vi "DependencyChecker.vi"() -> ()   [LabVIEW 2020]
uses:
  <vilib>/Utility/lvfile.llb/LVFileType.ctl
  FileDependencyType.ctl
  <vilib>/Utility/lvfile.llb/FT_FileTypes.ctl
  <vilib>/Utility/lvfile.llb/NI_FileType.lvlib
panel:
  out "size(s)":i32
  out "Files":map{path, T1}(c390)
  out "File Path 2":path
  out "Linker:Read Info From File":T4(array[cluster])
  in  "File Path":path=path "C:/Projects/DesignPatterns/Decorator1"
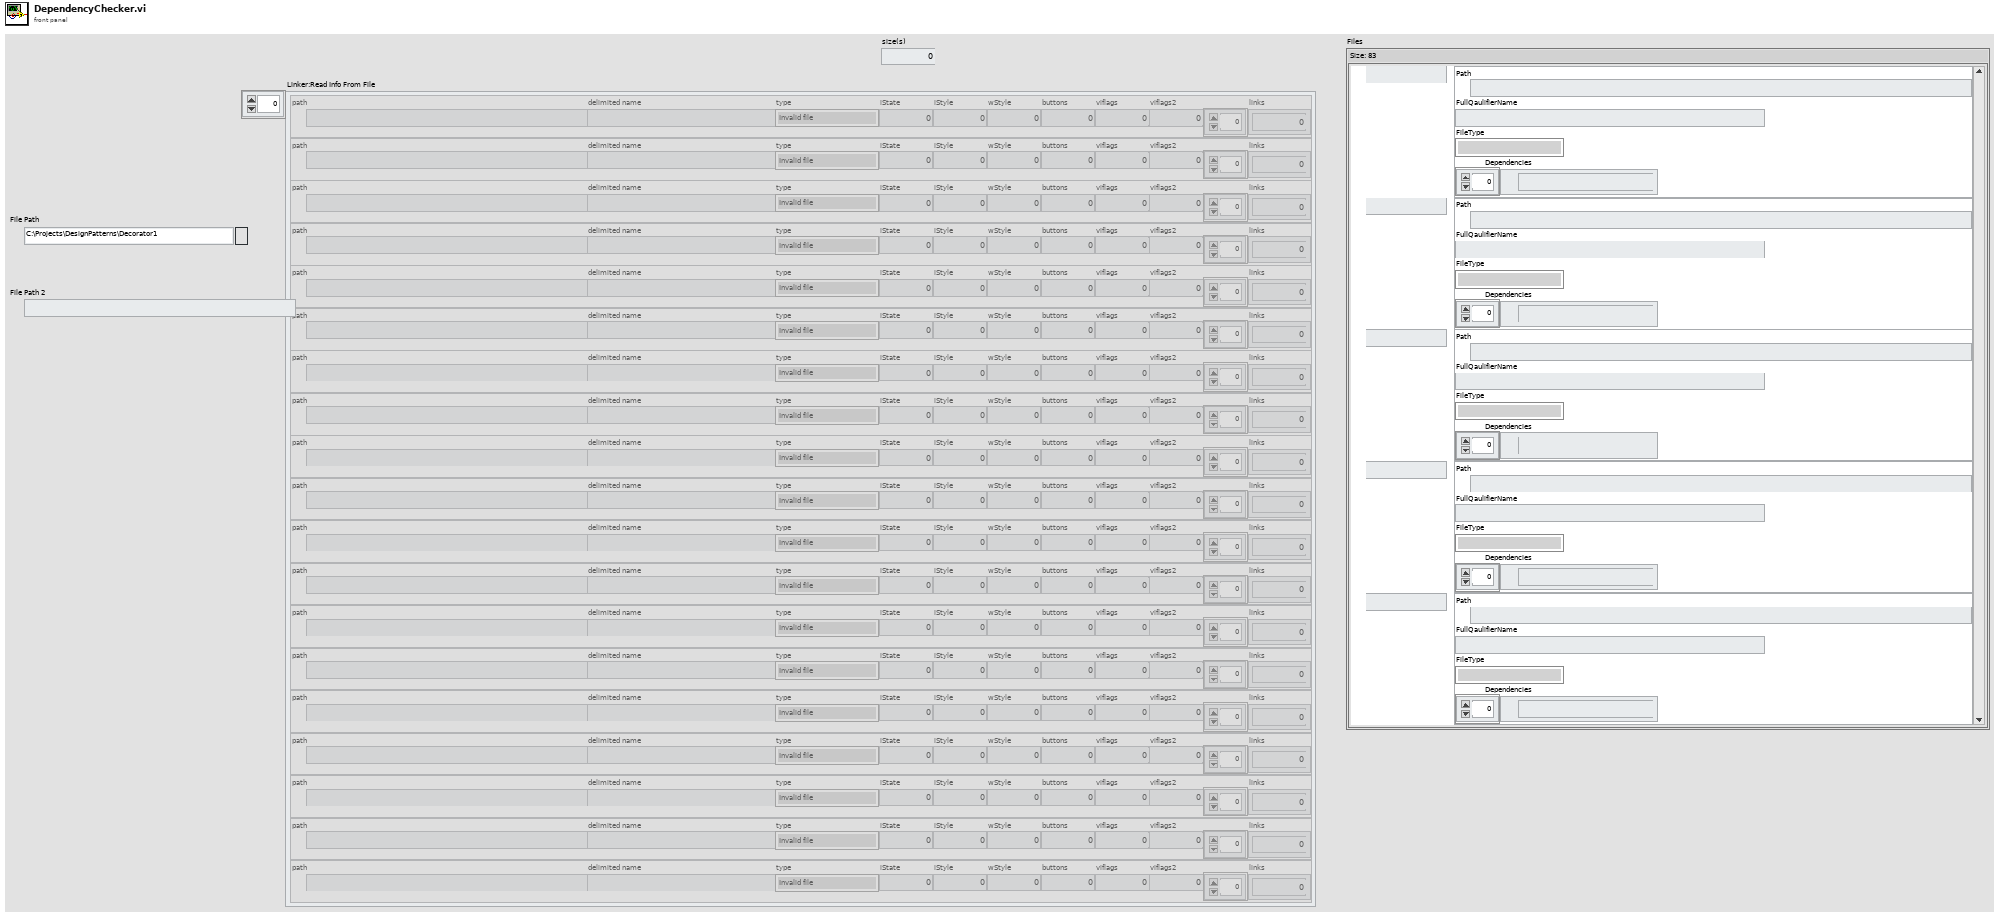
[diagram p1: front panel]
types:
  T1 = typedef "FileDependencyType.ctl" = cluster{"Path":path, "FullQaulifierName":string, "FileType":T2, "Dependencies":path[]}
  T2 = typedef "NI_FileType.lvlib/FT_FileTypes.ctl" = enum32{"Invalid file/path", "Unknown type", "Instrument", "Control", "Polymorphic VI", "Project", "Library", "LVClass", "XControl", "XNode", "CIN", "Run-time menu", "Palette menu", "LLB", "Shortcut", "Directory", "Class Private Data Control", "Statechart", "MathScript .m file", "Ladder Diagram", "LVLibp"}
  T3 = typedef "NI_FileType.lvlib/LVFileType.ctl" = enum32{"Invalid file", "Unknown type", "Instrument", "Control", "Polymorphic VI", "Project", "Library", "LVClass", "XControl", "XNode", "Shared library", ".NET assembly", "ActiveX interface", "CIN", "Run-time menu", "Palette menu", "Help file", "LLB", "XNode Edit Dependency", "Class Private Data Control", "Statechart", "MathScript .m file", "Ladder Diagram", "LVLibp", "XNode Build Dependency"}
  T4 = cluster{"path":path, "delimited name":string, "type":T3, "iState":u32, "iStyle":u16, "wStyle":u16, "buttons":u16, "viflags":u32, "viflags2":u32, "links":u32[]}[]
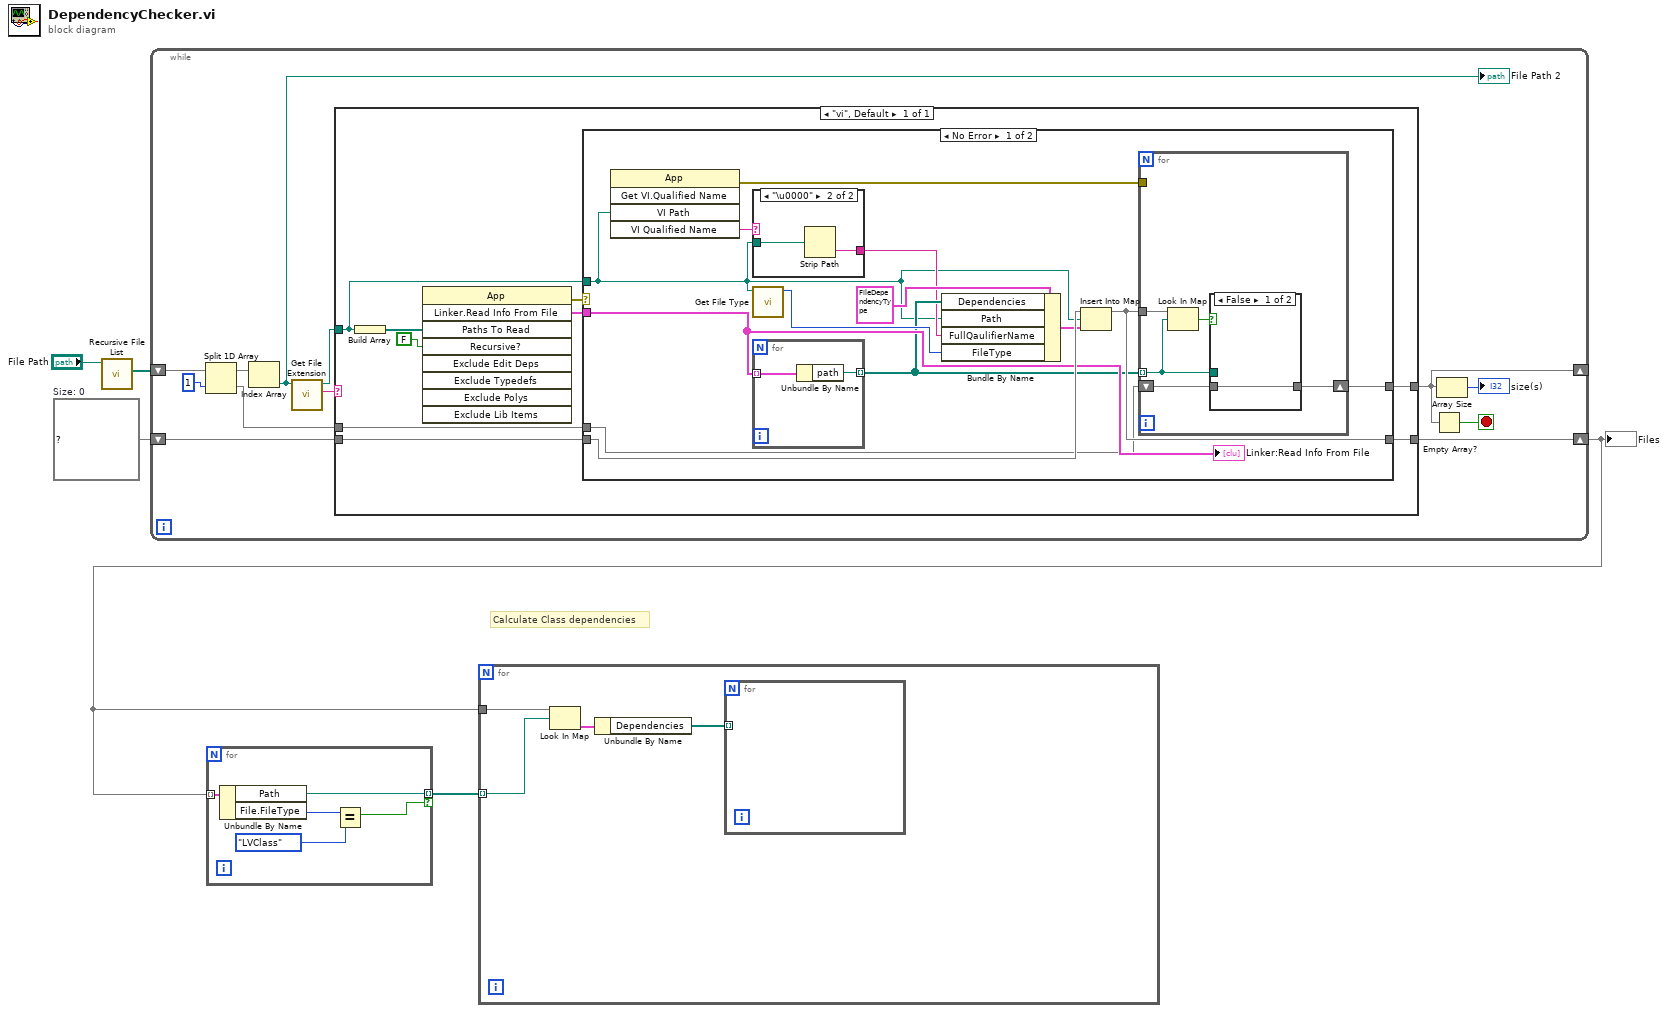
[diagram p0: block diagram]
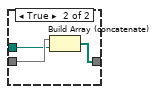
[diagram p3: hidden frame]
diagram:
  w3 = map{path, T1} {}  # Size: 0
  # "Calculate Class dependencies"
  n1 = call <vilib>:"Recursive File List.vi"("Folder Path"="File Path") -> ("All Files in Dir"=w4:path[])  [unwired: 6 in, 4 out]
  n2 = while {
    shift-right: [w9] -> w1
    shift-left: w3 -> [w15]
    shift-right: [w7] -> _
    shift-left: w4 -> [w14]
    stop <- w8 stop-if-true
    n3 = Split 1D Array(array=w14, index=1) -> (first subarray=w12:path[], second subarray=w10:path[])
    n4 = Index Array(array=w12) -> (element=w11:path)  [unwired: 1 in]
    "File Path 2" <- w11
    n5 = call <vilib>:"Get File Extension.vi"("file"=w11) -> ("lowercase file extension"=w17:string, "dup file"=w16:path)  [unwired: 6 in, 3 out]
    n6 = case shown="\"vi\", Default" w17 {
      tunnel: w16 -> [w19]
      tunnel: w15 -> [w22]
      tunnel: w10 -> [w21]
      tunnel: [w20] -> w7
      tunnel: [w18] -> w9
      frame "vi", Default {
        n7 = Build Array(w19) -> (w26:path[])
        n8 = invoke class="App" method="Linker.Read Info From File"("Paths To Read"=w26, "Recursive?"=FALSE) -> (error out=w23:errorcluster, "Linker.Read Info From File"=w24:T4)  [unwired: 7 in, 7 out]
        n9 = case shown="No Error" w23 {
          tunnel: w24 -> [w37 _]
          tunnel: w22 -> [w39 w54]
          tunnel: w21 -> [w32 w55]
          tunnel: [w31 w55] -> w20
          tunnel: w19 -> [w27 _]
          tunnel: [w34 w54] -> w18
          frame No Error {
            n10 = invoke class="App" method="Get VI.Qualified Name"("VI Path"=w27) -> (error out=w30:errorcluster, "VI Qualified Name"=w29:string)  [unwired: 4 in, 3 out]
            n11 = case shown="\"\"" w29 {
              selector: w29 -> [w40 _]
              tunnel: [w40 w41] -> w28
              tunnel: w27 -> [_ w42]
              frame Default {
              }
              frame "\u0000" {
                n12 = Strip Path(path=w42) -> (name=w41:string)  [unwired: 1 out]
              }
            }
            n13 = call <vilib>:"Get File Type.vi"("path"=w27) -> ("file type"=w35:T2)  [unwired: 8 in, 2 out]
            n14 = for {
              tunnel: w37 -> [w53] mode=indexing
              tunnel: [w52] -> w33 mode=indexing
              n15 = Unbundle By Name(w53) -> ("path"=w52:path)
            }
            n16 = Bundle By Name(cluster=T1 {"Path"=path "", "FullQaulifierName"="Decorator1_Main.vi", "FileType"=enum."Instrument", "Dependencies"=[]} ("value"), "Dependencies"=w33, "Path"=w27, "FullQaulifierName"=w28, "FileType"=w35) -> (w36:T1)
            n17 = Insert Into Map(map in=w39, key=w27, value=w36) -> (map out=w34:map{path, T1})  [unwired: 2 out]
            n18 = for {
              tunnel: w34 -> [w47]
              tunnel: w33 -> [w43] mode=indexing
              shift-right: [w44] -> w31
              shift-left: w32 -> [w45]
              tunnel: w30 -> [_]
              n19 = Look In Map(map=w47, key=w43) -> (key not found?=w46:bool)  [unwired: 1 in, 1 out]
              n20 = case shown="False" w46 {
                tunnel: w45 -> [w48 w51]
                tunnel: [w48 w50] -> w44
                tunnel: w43 -> [_ w49]
                frame False {
                }
                frame True {
                  n21 = Build Array (concatenate)(w51, w49) -> (w50:path[])
                }
              }
            }
            "Linker:Read Info From File" <- w37
          }
          frame Error {
          }
        }
      }
    }
    n22 = Empty Array?(array=w7) -> (empty?=w8:bool)
    n23 = Array Size(array=w7) -> (size(s)=→"size(s)":i32)
  }
  "Files" <- w1
  n24 = for {
    tunnel: w1 -> [w60] mode=indexing
    tunnel: [w57] -> w2 mode=indexing if=w56
    n25 = Unbundle By Name(w60) -> ("Path"=w57:path, "File.FileType"=w59:T2)
    n26 = Equal?(x=w59, y=FT_FileTypes."LVClass") -> (x = y?=w56:bool)
  }
  n27 = for {
    tunnel: w2 -> [w63] mode=indexing
    tunnel: w1 -> [w64]
    n28 = Look In Map(map=w64, key=w63) -> (value=w62:T1)  [unwired: 1 in, 1 out]
    n29 = Unbundle By Name(w62) -> ("Dependencies"=w61:path[])
    n30 = for {
      tunnel: w61 -> [_] mode=indexing
    }
  }
